vi "readLabelTypeForH3C.vi"(0 "input_str_labelType":string) -> (1 "show_str_011string":string, 2 "show_str_QSFP+?":string)   [LabVIEW 2011]
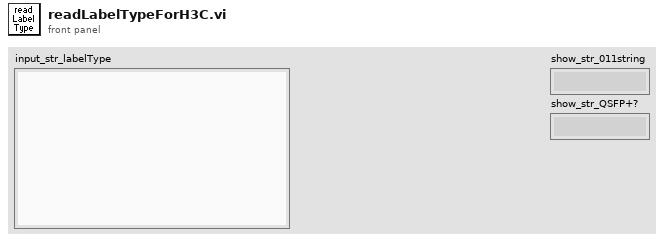
[diagram p1: front panel]
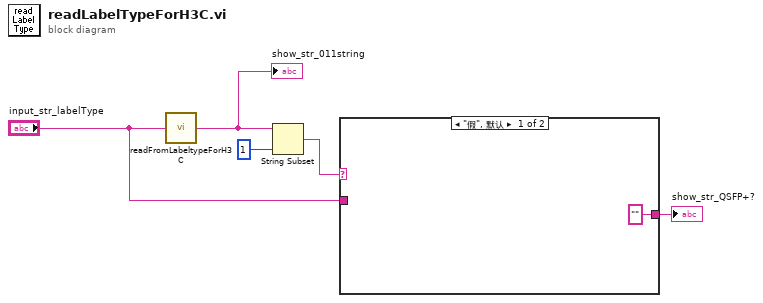
[diagram p0: block diagram]
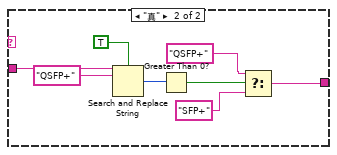
[diagram p2: hidden frame]
diagram:
  n1 = call "readFromLabeltypeForH3C.vi"("input_str_labelType"="input_str_labelType") -> ("show_str_011string"=w5:string)
  "show_str_011string" <- w5
  n2 = String Subset(string=w5, length (rest)=1 ("长度（剩余）")) -> (substring=w3:string)  [unwired: 1 in]
  n3 = case shown="\"假\", 默认" w3 {
    tunnel: "input_str_labelType" -> [_ w14]
    tunnel: ["" ("搜索字符串") w7] -> w1
    frame "假", Default {
    }
    frame "真" {
      n4 = Search and Replace String(case sensitive?=TRUE ("忽略大小写？(F)"), input string=w14, search string="QSFP+" ("搜索字符串")) -> (number of replacements=w11:i32)  [unwired: 5 in, 3 out]
      n5 = Greater Than 0?(x=w11) -> (x > 0?=w10:bool)
      n6 = Select(t="QSFP+" ("搜索字符串"), s=w10, f="SFP+" ("搜索字符串")) -> (s? t:f=w7:string)
    }
  }
  "show_str_QSFP+?" <- w1
